vi "Configure.vi"(5 "Experimenter":string(combo)="Unselected", 7 "Subject":string(combo)="Testing", 8 "error in (no error)":errorcluster, 9 "Sample Lines":tag[](array[tag])=["/Dev1/PFI0", "/Dev1/PFI1", "/Dev1/PFI2", "/Dev1/PFI3", "/Dev1/PFI4", "/Dev1/PFI5", "/Dev1/PFI6", "/Dev1/PFI7"], 10 "DAQmx Device Name":tag="6608", 11 "TimeStamper in":refnum<class "TimeStamper.lvclass">) -> (0 "error out":errorcluster, 3 "TimeStamper out":refnum<class "TimeStamper.lvclass">)   [LabVIEW 2010, in "TimeStamper.lvclass"]
uses:
  TimeStamper.lvclass
  TimeStamper.lvclass/TimeStamper.ctl
  <vilib>/Utility/config.llb/Read Key (I32).vi
  <vilib>/DAQmx/create/channels.llb/DAQmx Create Channel (CI-Count Edges).vi
  <vilib>/DAQmx/configure/timing.llb/DAQmx Timing (Sample Clock).vi
  Program Files/National Instruments/LabVIEW 2010/resource/objmgr/daqmx.rc
  <vilib>/Utility/config.llb/NI_LVConfig.lvlib
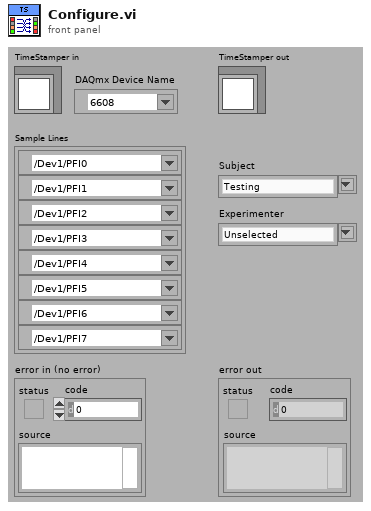
[diagram p1: front panel]
types:
  T1 = typedef "NI_LVConfig.lvlib/Config Data RefNum.ctl" = refnum<k1>
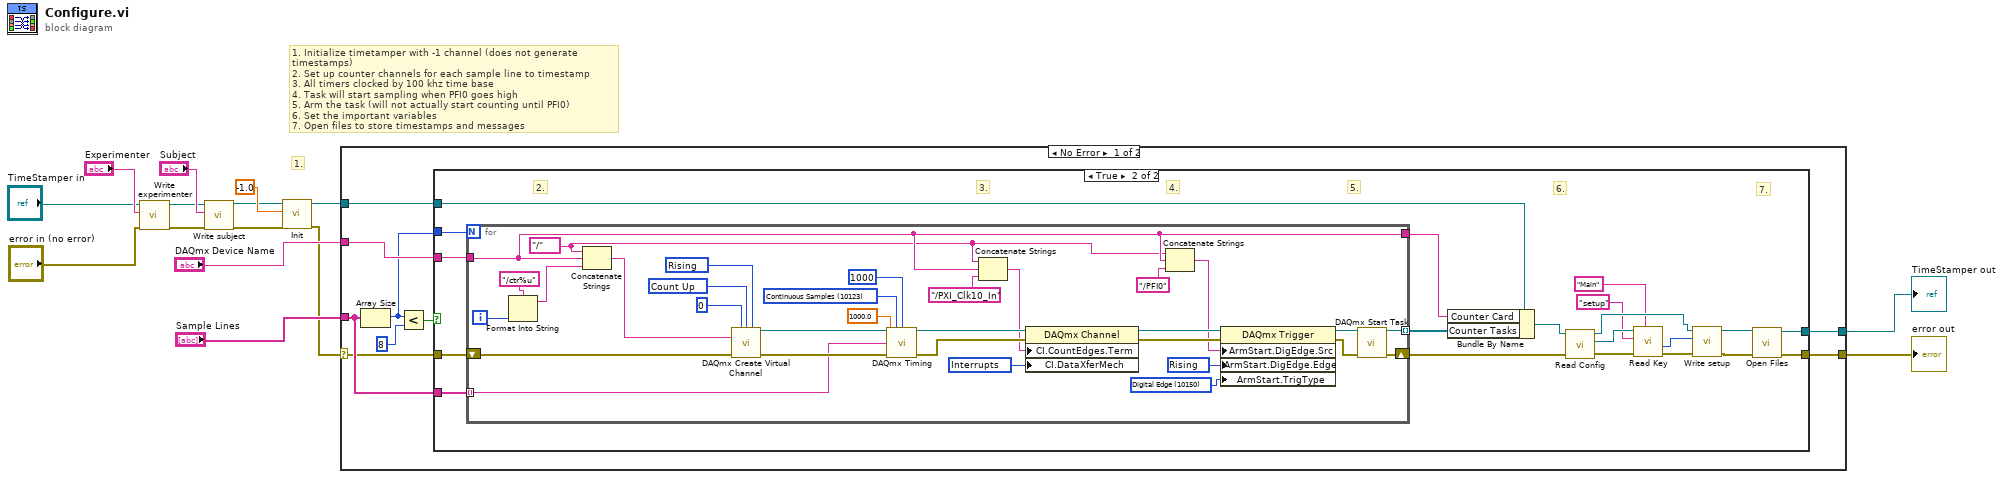
[diagram p0: block diagram]
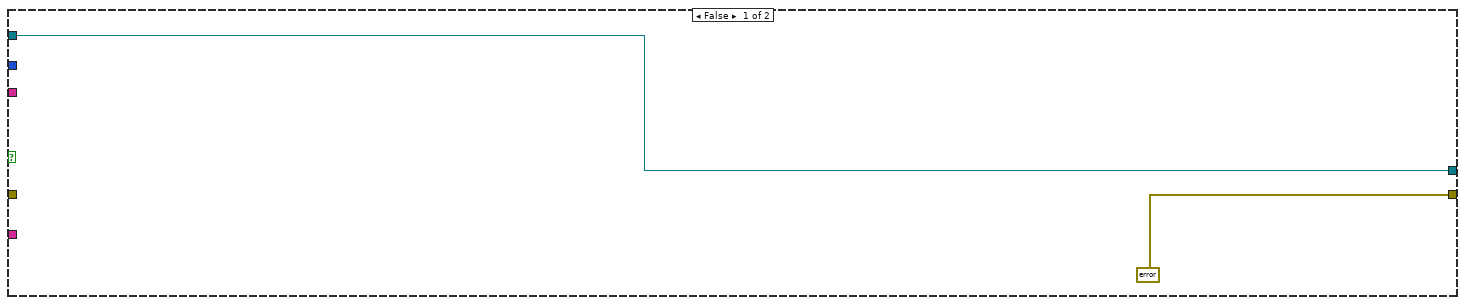
[diagram p2: hidden frame]
diagram:
  # "1. Initialize timetamper with -1 channel (does not generate timestamps)\n2. Set up counter channels for each sample line to timestamp\n3. All timers clocked by 100 khz time base\n4. Task will start sampling when PFI0 goes high\n5. Arm the task (will not actually start counting until PFI0)\n6. Set the important variables\n7. Open files to store timestamps and messages"
  # "1."
  n1 = call-dynamic "Write experimenter.vi"("error in (no error)"="error in (no error)", "experimenter"="Experimenter", "TimeStamper in"="TimeStamper in") -> ("error out"=w5:errorcluster, "TimeStamper out"=w6:refnum<class "TimeStamper.lvclass">)  [unwired: 7 in]
  n2 = call-dynamic "Write subject.vi"("error in (no error)"=w5, "subject"="Subject", "TimeStamper in"=w6) -> ("error out"=w4:errorcluster, "TimeStamper out"=w3:refnum<class "TimeStamper.lvclass">)  [unwired: 7 in]
  n3 = call-dynamic "Init.vi"("error in (no error)"=w4, "Channel"=-1.0, "AcquistionObject in"=w3) -> ("error out"=w11:errorcluster, "AcquistionObject out"=w9:refnum<class "TimeStamper.lvclass">)  [unwired: 7 in]
  n4 = case shown="No Error" w11 {
    selector: w11 -> [w19 w79]
    tunnel: [w18 w79] -> w15
    tunnel: [w16 w78] -> w14
    tunnel: w9 -> [w17 w78]
    tunnel: "Sample Lines" -> [w20 _]
    tunnel: "DAQmx Device Name" -> [w22 _]
    frame No Error {
      n5 = Array Size(array=w20) -> (size(s)=w21:i32)
      n6 = Less?(x=w21, y=8) -> (x < y?=w23:bool)
      n7 = case shown="True" w23 {
        tunnel: w22 -> [_ w41]
        tunnel: w21 -> [_ w46]
        tunnel: w20 -> [_ w45]
        tunnel: w19 -> [_ w44]
        tunnel: [errorcluster {"status"=TRUE, "code"=-150, "source"="Cannot initialize that many timestamped lines."} ("error IO") w39] -> w18
        tunnel: w17 -> [w26 w43]
        tunnel: [w26 w38] -> w16
        frame False {
        }
        frame True {
          # "6."
          # "7."
          # "5."
          # "4."
          # "3."
          # "2."
          n8 = for {
            N: w46 -> [_]
            tunnel: w41 -> [w50]
            tunnel: w45 -> [w57] mode=indexing
            shift-right: [w47] -> w30
            shift-left: w44 -> [w56]
            tunnel: [w55] -> w42 mode=indexing
            tunnel: [w50] -> w40
            i -> [w76]
            w49 = tag "/" ("string")
            w59 = 10204 items=["DMA"=10054, "Interrupts"=10204, "Programmed I/O"=10264, "USB Bulk"=12590] ("CI.DataXferMech")
            w60 = 10150 items=["Digital Edge"=10150, "None"=10230] ("ArmStart.TrigType")
            w61 = 10280 items=["Rising"=10280, "Falling"=10171] ("ArmStart.DigEdge.Edge")
            w69 = 10123 items=["Finite Samples"=10178, "Continuous Samples"=10123, "Hardware Timed Single Point"=12522] ("sample mode")
            w72 = 10280 items=["Rising"=10280, "Falling"=10171] ("edge")
            w73 = 10128 items=["Count Up"=10128, "Count Down"=10124, "Externally Controlled"=10326] ("count direction")
            n9 = Format Into String(format string="/ctr%u", w76) -> (resulting string=w75:string)  [unwired: 2 in, 1 out]
            n10 = Concatenate Strings(w49, w50, w75) -> (w58:string)
            n11 = call-poly <vilib>:"DAQmx Create Virtual Channel.vi"("initial count"=0, "count direction"=w73, "edge"=w72, "counter"=w58, "error in"=w56) -> ("task out"=w71:refnum<k21>, "error out"=w70:errorcluster)  [unwired: 9 in]
            n12 = call-poly <vilib>:"DAQmx Timing.vi"("task/channels in"=w71, "sample mode"=w69, "samples per channel"=1000, "rate"=1000.0, "source"=w57, "error in"=w70) -> ("task out"=w64:refnum<k21>, "error out"=w65:errorcluster)  [unwired: 8 in]
            n13 = Concatenate Strings(w49, w50, "/PXI_Clk10_In" ("string")) -> (w53:string)
            n14 = property class="DAQmx Channel"(reference=w64, error in=w65, "CI.CountEdges.Term"=w53, "CI.DataXferMech"=w59) -> (reference out=w63:refnum<k21>, error out=w62:errorcluster)
            n15 = Concatenate Strings(w49, w50, "/PFI0" ("string")) -> (w51:string)
            n16 = property class="DAQmx Trigger"(reference=w63, error in=w62, "ArmStart.DigEdge.Src"=w51, "ArmStart.DigEdge.Edge"=w61, "ArmStart.TrigType"=w60) -> (reference out=w66:refnum<k21>, error out=w48:errorcluster)
            n17 = call <vilib>:"DAQmx Start Task.vi"("task/channels in"=w66, "error in"=w48) -> ("task out"=w55:refnum<k21>, "error out"=w47:errorcluster)  [unwired: 12 in]
          }
          n18 = Bundle By Name(cluster=w43, "Counter Card"=w40, "Counter Tasks"=w42) -> (w29:refnum<class "TimeStamper.lvclass">)
          n19 = call-dynamic "Read Config.vi"("error in (no error)"=w30, "AcquistionObject in"=w29) -> ("error out"=w34:errorcluster, "config data"=w33:T1, "AcquistionObject out"=w37:refnum<class "TimeStamper.lvclass">)  [unwired: 7 in]
          n20 = call-poly <vilib>:"Read Key.vi"("section"="Main", "error in (no error)"=w34, "key"="setup", "refnum"=w33) -> ("error out"=w35:errorcluster, "value"=w36:i32)  [unwired: 4 in, 2 out]
          n21 = call-dynamic "Write setup.vi"("error in (no error)"=w35, "setup"=w36, "TimeStamper in"=w37) -> ("error out"=w27:errorcluster, "TimeStamper out"=w28:refnum<class "TimeStamper.lvclass">)  [unwired: 7 in]
          n22 = call-dynamic "Open Files.vi"("error in (no error)"=w27, "TimeStamper in"=w28) -> ("error out"=w39:errorcluster, "TimeStamper out"=w38:refnum<class "TimeStamper.lvclass">)  [unwired: 8 in]
        }
      }
    }
    frame Error {
    }
  }
  "error out" <- w15
  "TimeStamper out" <- w14
